vi "AssertConnectorPanesMatchExpected.vi"(8 "error in (no error)":errorcluster, 10 "custom device xml path":path, 11 "TestCase in":refnum<class "TestCase.lvclass">) -> (0 "error out":errorcluster, 3 "TestCase out":refnum<class "TestCase.lvclass">)   [LabVIEW 2015, in "VeriStandTestCase.lvclass"]
uses:
  VeriStandTestCase.lvclass
  <vilib>/addons/_JKI Toolkits/VI Tester/TestCase.llb/TestCase.lvclass
  Utilities/ConnectorPaneTemplate.ctl
  <userlib>/_OpenG.lib/file/file.llb/Append Path to Root if Relative - Scalar__ogtk.vi
panel:
  in  "connector pane templates":T1[](array[typedef])=[{"Template File"=path "NI Veristand/Custom Device API/ActionVIOnCompile Template.vit", "XPath Key"="//ActionVIOnCompile/Path/text()"}, {"Template File"=path "NI Veristand/Custom Device API/ActionVIOnDelete Template.vit", "XPath Key"="//ActionVIOnDelete/Path/text()"}, {"Template File"=path "NI Veristand/Custom Device API/ActionVIOnDeleteRequested Template.vit", "XPath Key"="//ActionVIOnDeleteRequested/Path/text()"}, {"Template File"=path "NI Veristand/Custom Device API/ActionVIOnDownload.vit", "XPath Key"="//ActionVIOnDownload/Path/text()"}, {"Template File"=path "NI Veristand/Custom Device API/ActionVIOnLoad Template.vit", "XPath Key"="//ActionVIOnLoad/Path/text()"}, {"Template File"=path "NI Veristand/Custom Device API/ActionVIOnPaste Template.vit", "XPath Key"="//ActionVIOnPaste/Path/text()"}, {"Template File"=path "NI Veristand/Custom Device API/ActionVIOnSave Template.vit", "XPath Key"="//ActionVIOnSave/Path/text()"}, {"Template File"=path "NI Veristand/Custom Device API/ActionVIOnShutdown Template.vit", "XPath Key"="//ActionVIOnShutdown/Path/text()"}, {"Template File"=path "NI Veristand/Custom Device API/Page Template.vit", "XPath Key"="//Page/Item2Launch/Path/text()"}, {"Template File"=path "NI Veristand/Custom Device API/Initialization VI Template.vit", "XPath Key"="//InitializationVI/Item2Launch/Path/text()"}, {"Template File"=path "NI Veristand/Custom Device API/RunTimeMenu Custom Item 2 Launch.vit", "XPath Key"="//RunTimeMenu/MenuItem[Type=\"Action\"]/Item2Launch/Path/text()"}, {"Template File"=path "NI Veristand/Custom Device API/Timing Source Initialization VI Template.vit", "XPath Key"="//TimingSource//RealTimeSystemDestination/text()"}]
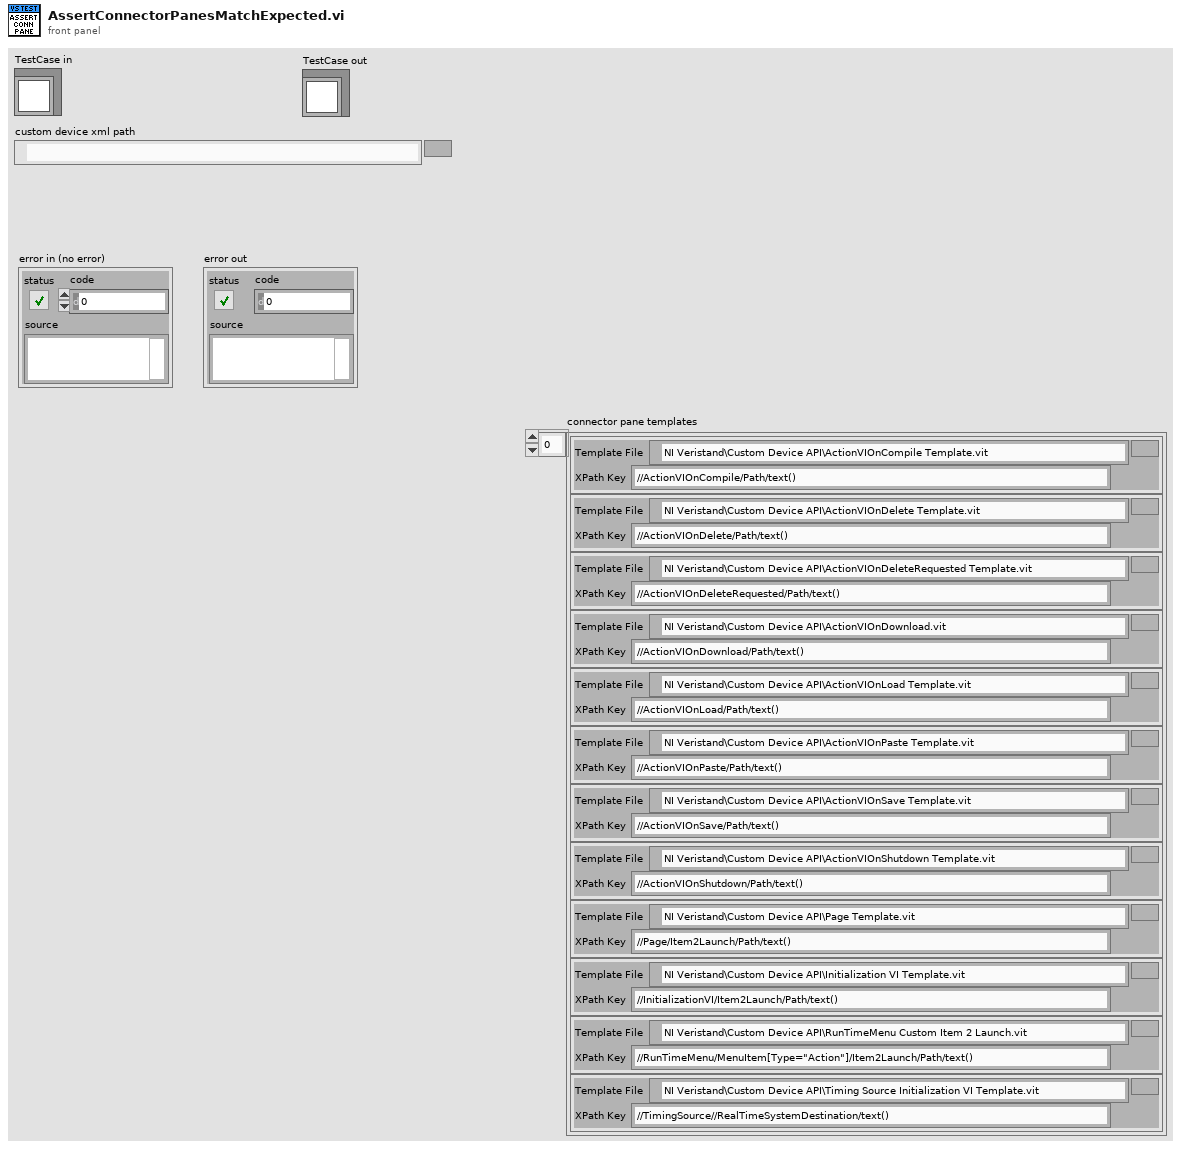
[diagram p1: front panel]
types:
  T1 = typedef "VeriStandTestCase.lvclass/ConnectorPaneTemplate.ctl" = cluster{"Template File":path, "XPath Key":string}
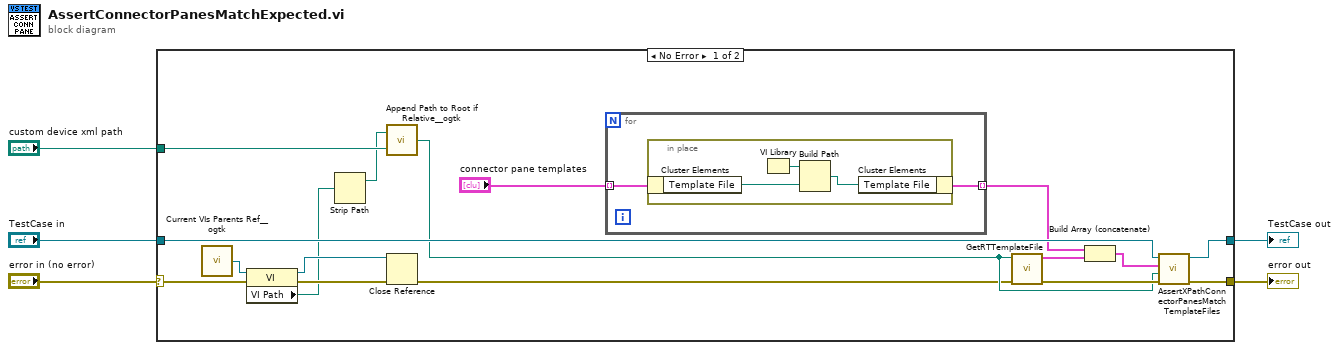
[diagram p0: block diagram]
diagram:
  n1 = case shown="No Error" "error in (no error)" {
    selector: "error in (no error)" -> [w8 w29]
    tunnel: [w21 w29] -> w5
    tunnel: "custom device xml path" -> [w22 _]
    tunnel: "TestCase in" -> [w19 w28]
    tunnel: [w20 w28] -> w1
    frame No Error {
      n2 = call <userlib>:"Current VIs Parents Ref__ogtk.vi"() -> ("Calling VI's Reference"=w12:refnum<vi>)  [unwired: 2 in]
      n3 = property class="VI"(reference=w12, error in=w8) -> (reference out=w11:refnum<vi>, error out=w10:errorcluster, "VI Path"=w6:path)
      n4 = Strip Path(path=w6) -> (stripped path=w7:path)  [unwired: 1 out]
      n5 = call-poly <userlib>:"Append Path to Root if Relative__ogtk.vi"("Absolute or Relative Path"=w22, "Root Path"=w7) -> ("Absolute or Appended Path"=w13:path)
      n6 = Close Reference(reference=w11, error in (no error)=w10) -> (error out=w9:errorcluster)
      n7 = for {
        tunnel: "connector pane templates" -> [w24] mode=indexing
        tunnel: [w23] -> w14 mode=indexing
        n8 = in-place {
          n9 = in-place-cluster #1(w24) -> ("Template File"=w25:path)
          n10 = VI Library() -> (path=w27:path)
          n11 = Build Path(base path=w27, name or relative path=w25) -> (appended path=w26:path)
          n12 = in-place-cluster #1("Template File"=w26) -> (w23:T1)
        }
      }
      n13 = call "GetRTTemplateFile.vi"("error in (no error)"=w9, "absolute custom device xml file"=w13) -> ("error out"=w18:errorcluster, "connector pane template"=w17:T1)  [unwired: 8 in]
      n14 = Build Array (concatenate)(w14, w17) -> (w16:T1[])
      n15 = call "AssertXPathConnectorPanesMatchTemplateFiles.vi"("error in (no error)"=w18, "absolute custom device xml file"=w13, "connector pane templates"=w16, "TestCase in"=w19) -> ("error out"=w21:errorcluster, "TestCase out"=w20:refnum<class "TestCase.lvclass">)  [unwired: 6 in]
    }
    frame Error {
    }
  }
  "error out" <- w5
  "TestCase out" <- w1
